vi "DSF.Engine.Sequencer Bundle.Set Iteration.vi"(8 "error in (no error)":errorcluster, 10 "iteration":u64, 11 "Sequencer Bundle in":refnum<class "DSF.Engine.Sequencer.Timing Bundle.lvclass">) -> (0 "error out":errorcluster, 3 "Sequencer Bundle out":refnum<class "DSF.Engine.Sequencer.Timing Bundle.lvclass">)   [LabVIEW 2017, in "DSF.Engine.lvlib" / "DSF.Engine.Sequencer.Timing Bundle.lvclass"]
uses:
  DSF.Engine.Sequencer.Timing Bundle.lvclass
  DSF.Engine.Sequencer.Timing Bundle.lvclass/DSF.Engine.Sequencer.Timing Bundle.ctl
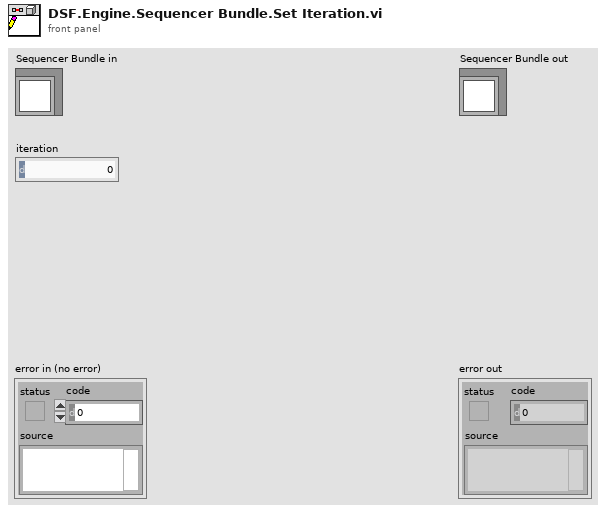
[diagram p1: front panel]
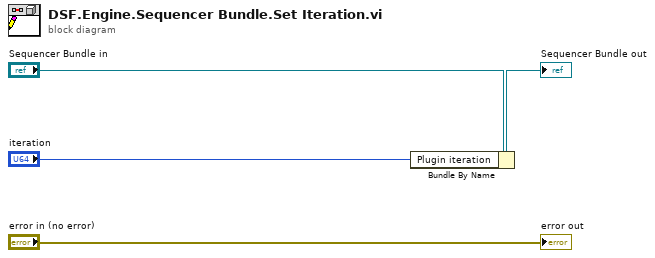
[diagram p0: block diagram]
diagram:
  n1 = Bundle By Name(cluster="Sequencer Bundle in", "Plugin iteration"="iteration") -> (→"Sequencer Bundle out":refnum<class "DSF.Engine.Sequencer.Timing Bundle.lvclass">)
  "error out" <- "error in (no error)"
